vi "输入数据解析.vi"(0 "单个参数补充":dbl, 1 "从板号":dbl=1.0, 2 "主板二维码":string="BNET01", 3 "从板二维码":string="BNET01", 5 "主板引用":refnum<vi>, 7 "从板引用":refnum<vi>, 9 "主板选项":string="三级故障阀值", 11 "枚举":enum16{"主板", "从板"}(ring), 12 "快换":bool caption="快换写入") -> (4 "输出数组":dbl[][](array[numeric]), 6 "数组长度":dbl[](array[numeric]), 8 "循环次数":i32, 10 "命令":u32, 14 "名称":string[](array[string]), 15 "命令序号":u32[](array[numeric]))   [LabVIEW 2013] (continued)
                n1310 = Build Array(w3277) -> (w3278:i32[])
              }
              frame 16 {
                # "SOH过低"
                n1311 = disable-structure shown="启用" {
                  disable-tunnel: [w3302 w3310] -> w3289
                  disable-tunnel: w3288 -> [w3299 _]
                  disable-tunnel: [w3291 w3310] -> w3287
                  frame Disabled {
                    n1312 = Unbundle By Name(w3299) -> ("SOH过低"=w3298:dbl)
                    n1313 = call "输入分辨率计算-EV05.vi"("1字节?"=FALSE, "数值"=w3298, "偏移量"=0.0, "分辨率"=0.1) -> ("低字节"=w3300:dbl, "高字节1"=w3301:dbl)  [unwired: 1 in, 5 out]
                    n1314 = call "二进制解析-8.6.vi"("索引"=4, "数值"=w3301) -> ("低位子数组"=w3304:i32[])  [unwired: 3 out]
                    n1315 = call "二进制解析-8.6.vi"("索引"=4, "数值"=w3300) -> ("低位子数组"=w3293:i32[], "高位子数组"=w3303:i32[])  [unwired: 2 out]
                    n1316 = call "二进制解析-8.6.vi"("索引"=4, "数值"=0) -> ("低位子数组"=w3294:i32[])  [unwired: 3 out]
                    n1317 = Insert Into Array(array=w3304, new element=w3303) -> (w3297:i32[])  [unwired: 1 in]
                    n1318 = Insert Into Array(array=w3293, new element=w3294) -> (w3292:i32[])  [unwired: 1 in]
                    n1319 = call "数值二进制转十进制-8.6.vi"("子数组"=w3297) -> ("十进制数值"=w3302:i32)  [unwired: 4 out]
                    n1320 = call "数值二进制转十进制-8.6.vi"("子数组"=w3292) -> ("十进制数值"=w3291:i32)  [unwired: 4 out]
                  }
                  frame Enabled {
                    w3310 = 255 ("高字节1")
                  }
                }
                n1321 = Build Array(w3289, w3287) -> (w3290:i32[])
              }
            }
            n1322 = Insert Into Array(array=w3094, new element=w3095) -> (w3093:dbl[])  [unwired: 1 in]
          }
          n1323 = Build Array(w3090) -> (w3089:dbl[][])
          n1324 = Build Array("一级故障阀值") -> (w3080:string[])
        }
        frame "温度过低(2)" {
          n1325 = Unbundle By Name(w3316) -> ("一级故障 2"=w3317:refnum<vi>)
          n1326 = property class="Clust (严格)"(reference=w3317) -> ("Value"=w3315:T4)  [unwired: 1 in, 2 out]
          n1327 = for {
            N: 17 -> [_]
            tunnel: w3315 -> [w3327]
            shift-right: [w3324] -> w3321
            shift-left: dbl[] [] -> [w3325]
            i -> [w3328]
            n1328 = case shown="13" w3328 {
              tunnel: w3327 -> [w3329 w3340 w3351 w3361 w3371 w3381 w3393 w3405 w3417 w3429 w3441 w3453 w3467 w3489 w3501 w3510 w3519]
              tunnel: [w3330 w3341 w3352 w3362 w3372 w3383 w3395 w3407 w3419 w3431 w3443 w3454 w3476 w3492 w3500 w3509 w3521] -> w3326
              frame 0, Default {
                # "总电压过高"
                n1329 = disable-structure shown="启用" {
                  disable-tunnel: [w3336 w3339] -> w3332
                  disable-tunnel: [w3335 w3339] -> w3331
                  disable-tunnel: w3329 -> [w3334 _]
                  frame Disabled {
                    n1330 = Unbundle By Name(w3334) -> ("总电压过高"=w3333:dbl)
                    n1331 = call "输入分辨率计算-EV05.vi"("1字节?"=FALSE, "数值"=w3333, "分辨率"=0.1) -> ("低字节"=w3336:dbl, "高字节1"=w3335:dbl)  [unwired: 2 in, 5 out]
                  }
                  frame Enabled {
                    w3339 = 255 ("高字节1")
                  }
                }
                n1332 = Build Array(w3331, w3332) -> (w3330:i32[])
              }
              frame 1 {
                # "总电压过低"
                n1333 = disable-structure shown="启用" {
                  disable-tunnel: [w3347 w3350] -> w3343
                  disable-tunnel: [w3346 w3350] -> w3342
                  disable-tunnel: w3340 -> [w3345 _]
                  frame Disabled {
                    n1334 = Unbundle By Name(w3345) -> ("总电压过低"=w3344:dbl)
                    n1335 = call "输入分辨率计算-EV05.vi"("1字节?"=FALSE, "数值"=w3344, "分辨率"=0.1) -> ("低字节"=w3347:dbl, "高字节1"=w3346:dbl)  [unwired: 2 in, 5 out]
                  }
                  frame Enabled {
                    w3350 = 255 ("高字节1")
                  }
                }
                n1336 = Build Array(w3342, w3343) -> (w3341:i32[])
              }
              frame 2 {
                # "温度过高"
                n1337 = disable-structure shown="启用" {
                  disable-tunnel: [w3357 255 ("高字节1")] -> w3353
                  disable-tunnel: w3351 -> [w3355 _]
                  frame Disabled {
                    n1338 = Unbundle By Name(w3355) -> ("温度过高"=w3354:dbl)
                    n1339 = call "输入分辨率计算-EV05.vi"("1字节?"=TRUE, "数值"=w3354, "偏移量"=-40.0, "分辨率"=1.0) -> ("高字节1"=w3357:dbl)  [unwired: 1 in, 6 out]
                  }
                  frame Enabled {
                  }
                }
                n1340 = Build Array(w3353) -> (w3352:i32[])
              }
              frame 3 {
                # "温度过低"
                n1341 = disable-structure shown="启用" {
                  disable-tunnel: [w3367 255 ("高字节1")] -> w3363
                  disable-tunnel: w3361 -> [w3365 _]
                  frame Enabled {
                    n1342 = Unbundle By Name(w3365) -> ("温度过低"=w3364:dbl)
                    n1343 = call "输入分辨率计算-EV05.vi"("1字节?"=TRUE, "数值"=w3364, "偏移量"=-40.0, "分辨率"=1.0) -> ("高字节1"=w3367:dbl)  [unwired: 1 in, 6 out]
                  }
                  frame Disabled {
                  }
                }
                n1344 = Build Array(w3363) -> (w3362:dbl[])
              }
              frame 4 {
                # "整组温度不均衡"
                n1345 = disable-structure shown="启用" {
                  disable-tunnel: [w3377 255 ("高字节1")] -> w3373
                  disable-tunnel: w3371 -> [w3375 _]
                  frame Disabled {
                    n1346 = Unbundle By Name(w3375) -> ("整组温度不均衡"=w3374:dbl)
                    n1347 = call "输入分辨率计算-EV05.vi"("1字节?"=TRUE, "数值"=w3374, "偏移量"=0.0, "分辨率"=1.0) -> ("高字节1"=w3377:dbl)  [unwired: 1 in, 6 out]
                  }
                  frame Enabled {
                  }
                }
                n1348 = Build Array(w3373) -> (w3372:i32[])
              }
              frame 5 {
                # "单组电压不均衡"
                n1349 = disable-structure shown="启用" {
                  disable-tunnel: [w3389 w3392] -> w3384
                  disable-tunnel: [w3387 w3392] -> w3382
                  disable-tunnel: w3381 -> [w3386 _]
                  frame Disabled {
                    n1350 = Unbundle By Name(w3386) -> ("单组电压不均衡"=w3385:dbl)
                    n1351 = call "输入分辨率计算-EV05.vi"("1字节?"=FALSE, "数值"=w3385, "偏移量"=0.0, "分辨率"=0.001) -> ("低字节"=w3387:dbl, "高字节1"=w3389:dbl)  [unwired: 1 in, 5 out]
                  }
                  frame Enabled {
                    w3392 = 255 ("高字节1")
                  }
                }
                n1352 = Build Array(w3384, w3382) -> (w3383:i32[])
              }
              frame 6 {
                # "整组电压不均衡"
                n1353 = disable-structure shown="启用" {
                  disable-tunnel: [w3401 w3404] -> w3396
                  disable-tunnel: [w3399 w3404] -> w3394
                  disable-tunnel: w3393 -> [w3398 _]
                  frame Disabled {
                    n1354 = Unbundle By Name(w3398) -> ("整组电压不均衡"=w3397:dbl)
                    n1355 = call "输入分辨率计算-EV05.vi"("1字节?"=FALSE, "数值"=w3397, "偏移量"=0.0, "分辨率"=0.001) -> ("低字节"=w3399:dbl, "高字节1"=w3401:dbl)  [unwired: 1 in, 5 out]
                  }
                  frame Enabled {
                    w3404 = 255 ("高字节1")
                  }
                }
                n1356 = Build Array(w3396, w3394) -> (w3395:i32[])
              }
              frame 7 {
                # "单体电压过高"
                n1357 = disable-structure shown="启用" {
                  disable-tunnel: [w3413 w3416] -> w3408
                  disable-tunnel: [w3411 w3416] -> w3406
                  disable-tunnel: w3405 -> [w3410 _]
                  frame Disabled {
                    n1358 = Unbundle By Name(w3410) -> ("单体电压过高"=w3409:dbl)
                    n1359 = call "输入分辨率计算-EV05.vi"("1字节?"=FALSE, "数值"=w3409, "偏移量"=0.0, "分辨率"=0.001) -> ("低字节"=w3411:dbl, "高字节1"=w3413:dbl)  [unwired: 1 in, 5 out]
                  }
                  frame Enabled {
                    w3416 = 255 ("高字节1")
                  }
                }
                n1360 = Build Array(w3408, w3406) -> (w3407:i32[])
              }
              frame 8 {
                # "单体电压过低"
                n1361 = disable-structure shown="启用" {
                  disable-tunnel: [w3425 w3428] -> w3420
                  disable-tunnel: [w3423 w3428] -> w3418
                  disable-tunnel: w3417 -> [w3422 _]
                  frame Disabled {
                    n1362 = Unbundle By Name(w3422) -> ("单体电压过低"=w3421:dbl)
                    n1363 = call "输入分辨率计算-EV05.vi"("1字节?"=FALSE, "数值"=w3421, "偏移量"=0.0, "分辨率"=0.001) -> ("低字节"=w3423:dbl, "高字节1"=w3425:dbl)  [unwired: 1 in, 5 out]
                  }
                  frame Enabled {
                    w3428 = 255 ("高字节1")
                  }
                }
                n1364 = Build Array(w3420, w3418) -> (w3419:i32[])
              }
              frame 9 {
                # "充电电流过高"
                n1365 = disable-structure shown="启用" {
                  disable-tunnel: [w3437 w3440] -> w3432
                  disable-tunnel: [w3435 w3440] -> w3430
                  disable-tunnel: w3429 -> [w3434 _]
                  frame Disabled {
                    n1366 = Unbundle By Name(w3434) -> ("充电电流过高"=w3433:dbl)
                    n1367 = call "输入分辨率计算-EV05.vi"("1字节?"=FALSE, "数值"=w3433, "偏移量"=-3000.0, "分辨率"=0.1) -> ("低字节"=w3435:dbl, "高字节1"=w3437:dbl)  [unwired: 1 in, 5 out]
                  }
                  frame Enabled {
                    w3440 = 255 ("高字节1")
                  }
                }
                n1368 = Build Array(w3432, w3430) -> (w3431:i32[])
              }
              frame 10 {
                # "放电电流过高"
                n1369 = disable-structure shown="启用" {
                  disable-tunnel: [w3449 w3452] -> w3444
                  disable-tunnel: [w3447 w3452] -> w3442
                  disable-tunnel: w3441 -> [w3446 _]
                  frame Disabled {
                    n1370 = Unbundle By Name(w3446) -> ("放电电流过高"=w3445:dbl)
                    n1371 = call "输入分辨率计算-EV05.vi"("1字节?"=FALSE, "数值"=w3445, "偏移量"=-3000.0, "分辨率"=0.1) -> ("低字节"=w3447:dbl, "高字节1"=w3449:dbl)  [unwired: 1 in, 5 out]
                  }
                  frame Enabled {
                    w3452 = 255 ("高字节1")
                  }
                }
                n1372 = Build Array(w3444, w3442) -> (w3443:i32[])
              }
              frame 11 {
                # "单组温度不均衡"
                n1373 = disable-structure shown="启用" {
                  disable-tunnel: [w3459 255 ("高字节1")] -> w3455
                  disable-tunnel: w3453 -> [w3457 _]
                  frame Disabled {
                    n1374 = Unbundle By Name(w3457) -> ("单组温度不均衡"=w3456:dbl)
                    n1375 = call "输入分辨率计算-EV05.vi"("1字节?"=TRUE, "数值"=w3456, "偏移量"=0.0, "分辨率"=1.0) -> ("高字节1"=w3459:dbl)  [unwired: 1 in, 6 out]
                  }
                  frame Enabled {
                  }
                }
                n1376 = Build Array(w3455) -> (w3454:i32[])
              }
              frame 12 {
                # "SOC过高"
                n1377 = Unbundle By Name(w3467) -> ("SOC过高"=w3466:dbl)
                n1378 = call "输入分辨率计算-EV05.vi"("1字节?"=FALSE, "数值"=w3466, "偏移量"=0.0, "分辨率"=0.1) -> ("低字节"=w3468:dbl, "高字节1"=w3469:dbl)  [unwired: 1 in, 5 out]
                n1379 = call "二进制解析-8.6.vi"("索引"=4, "数值"=w3469) -> ("低位子数组"=w3472:i32[])  [unwired: 3 out]
                n1380 = call "二进制解析-8.6.vi"("索引"=4, "数值"=w3468) -> ("低位子数组"=w3464:i32[], "高位子数组"=w3471:i32[])  [unwired: 2 out]
                n1381 = Insert Into Array(array=w3472, new element=w3471) -> (w3470:i32[])  [unwired: 1 in]
                n1382 = call "数值二进制转十进制-8.6.vi"("子数组"=w3470) -> ("十进制数值"=w3465:i32)  [unwired: 4 out]
                n1383 = disable-structure shown="启用" {
                  disable-tunnel: w3465 -> [w3480 _]
                  disable-tunnel: [w3480 255 ("高字节1")] -> w3463
                  disable-tunnel: [w3479 i32[] [] ("低位子数组 21")] -> _
                  disable-tunnel: w3464 -> [w3479 _]
                  frame Disabled {
                  }
                  frame Enabled {
                  }
                }
                n1384 = Build Array(w3463, w3463) -> (w3476:i32[])
              }
              frame 13 {
                # "SOC过低"
                n1385 = Unbundle By Name(w3489) -> ("SOC过低"=w3488:dbl)
                n1386 = call "输入分辨率计算-EV05.vi"("1字节?"=FALSE, "数值"=w3488, "偏移量"=0.0, "分辨率"=0.1) -> ("低字节"=w3486:dbl, "高字节1"=w3487:dbl)  [unwired: 1 in, 5 out]
                n1387 = call "二进制解析-8.6.vi"("索引"=4, "数值"=w3487) -> ("低位子数组"=w3484:i32[])  [unwired: 3 out]
                n1388 = disable-structure shown="启用" {
                  disable-tunnel: w3486 -> [w3496 _]
                  disable-tunnel: [w3496 255 ("高字节1")] -> w3485
                  disable-tunnel: w3484 -> [w3495 _]
                  disable-tunnel: [_ 255 ("高字节1")] -> w3483
                  frame Disabled {
                    (unwired) i32[] [] ("低位子数组 4")
                  }
                  frame Enabled {
                  }
                }
                n1389 = Build Array(w3483, w3485) -> (w3492:i32[])
              }
              frame 14 {
                # "内阻过大"
                n1390 = disable-structure shown="启用" {
                  disable-tunnel: w3501 -> [w3506 _]
                  disable-tunnel: [w3502 255 ("高字节1")] -> w3499
                  frame Disabled {
                    n1391 = Unbundle By Name(w3506) -> ("内阻过大"=w3505:dbl)
                    n1392 = call "输入分辨率计算-EV05.vi"("1字节?"=TRUE, "数值"=w3505, "分辨率"=0.1) -> ("高字节1"=w3502:dbl)  [unwired: 2 in, 6 out]
                  }
                  frame Enabled {
                  }
                }
                n1393 = Build Array(w3499) -> (w3500:i32[])
              }
              frame 15 {
                # "极柱温度过高"
                n1394 = disable-structure shown="启用" {
                  disable-tunnel: w3510 -> [w3516 _]
                  disable-tunnel: [w3512 255 ("高字节1")] -> w3508
                  frame Disabled {
                    n1395 = Unbundle By Name(w3516) -> ("极柱温度过高"=w3515:dbl)
                    n1396 = call "输入分辨率计算-EV05.vi"("1字节?"=TRUE, "数值"=w3515, "偏移量"=-40.0, "分辨率"=1.0) -> ("高字节1"=w3512:dbl)  [unwired: 1 in, 6 out]
                  }
                  frame Enabled {
                  }
                }
                n1397 = Build Array(w3508) -> (w3509:i32[])
              }
              frame 16 {
                # "SOH过低"
                n1398 = disable-structure shown="启用" {
                  disable-tunnel: [w3533 w3541] -> w3520
                  disable-tunnel: w3519 -> [w3530 _]
                  disable-tunnel: [w3522 w3541] -> w3518
                  frame Disabled {
                    n1399 = Unbundle By Name(w3530) -> ("SOH过低"=w3529:dbl)
                    n1400 = call "输入分辨率计算-EV05.vi"("1字节?"=FALSE, "数值"=w3529, "偏移量"=0.0, "分辨率"=0.1) -> ("低字节"=w3531:dbl, "高字节1"=w3532:dbl)  [unwired: 1 in, 5 out]
                    n1401 = call "二进制解析-8.6.vi"("索引"=4, "数值"=w3532) -> ("低位子数组"=w3535:i32[])  [unwired: 3 out]
                    n1402 = call "二进制解析-8.6.vi"("索引"=4, "数值"=w3531) -> ("低位子数组"=w3524:i32[], "高位子数组"=w3534:i32[])  [unwired: 2 out]
                    n1403 = call "二进制解析-8.6.vi"("索引"=4, "数值"=0) -> ("低位子数组"=w3525:i32[])  [unwired: 3 out]
                    n1404 = Insert Into Array(array=w3535, new element=w3534) -> (w3528:i32[])  [unwired: 1 in]
                    n1405 = Insert Into Array(array=w3524, new element=w3525) -> (w3523:i32[])  [unwired: 1 in]
                    n1406 = call "数值二进制转十进制-8.6.vi"("子数组"=w3528) -> ("十进制数值"=w3533:i32)  [unwired: 4 out]
                    n1407 = call "数值二进制转十进制-8.6.vi"("子数组"=w3523) -> ("十进制数值"=w3522:i32)  [unwired: 4 out]
                  }
                  frame Enabled {
                    w3541 = 255 ("高字节1")
                  }
                }
                n1408 = Build Array(w3520, w3518) -> (w3521:i32[])
              }
            }
            n1409 = Insert Into Array(array=w3325, new element=w3326) -> (w3324:dbl[])  [unwired: 1 in]
          }
          n1410 = Build Array(w3321) -> (w3320:dbl[][])
          n1411 = Build Array("二级故障阀值") -> (w3311:string[])
        }
        frame "温度过低(3)" {
          n1412 = Unbundle By Name(w3547) -> ("一级故障 3"=w3548:refnum<vi>)
          n1413 = property class="Clust (严格)"(reference=w3548) -> ("Value"=w3546:T4)  [unwired: 1 in, 2 out]
          n1414 = for {
            N: 17 -> [_]
            tunnel: w3546 -> [w3558]
            shift-right: [w3555] -> w3552
            shift-left: dbl[] [] -> [w3556]
            i -> [w3559]
            n1415 = case shown="13" w3559 {
              tunnel: w3558 -> [w3560 w3571 w3582 w3592 w3602 w3612 w3624 w3636 w3648 w3660 w3672 w3684 w3698 w3720 w3732 w3741 w3750]
              tunnel: [w3561 w3572 w3583 w3593 w3603 w3614 w3626 w3638 w3650 w3662 w3674 w3685 w3707 w3723 w3731 w3740 w3752] -> w3557
              frame 0, Default {
                # "总电压过高"
                n1416 = disable-structure shown="启用" {
                  disable-tunnel: [w3567 w3570] -> w3563
                  disable-tunnel: [w3566 w3570] -> w3562
                  disable-tunnel: w3560 -> [w3565 _]
                  frame Disabled {
                    n1417 = Unbundle By Name(w3565) -> ("总电压过高"=w3564:dbl)
                    n1418 = call "输入分辨率计算-EV05.vi"("1字节?"=FALSE, "数值"=w3564, "分辨率"=0.1) -> ("低字节"=w3567:dbl, "高字节1"=w3566:dbl)  [unwired: 2 in, 5 out]
                  }
                  frame Enabled {
                    w3570 = 255 ("高字节1")
                  }
                }
                n1419 = Build Array(w3562, w3563) -> (w3561:i32[])
              }
              frame 1 {
                # "总电压过低"
                n1420 = disable-structure shown="启用" {
                  disable-tunnel: [w3578 w3581] -> w3574
                  disable-tunnel: [w3577 w3581] -> w3573
                  disable-tunnel: w3571 -> [w3576 _]
                  frame Disabled {
                    n1421 = Unbundle By Name(w3576) -> ("总电压过低"=w3575:dbl)
                    n1422 = call "输入分辨率计算-EV05.vi"("1字节?"=FALSE, "数值"=w3575, "分辨率"=0.1) -> ("低字节"=w3578:dbl, "高字节1"=w3577:dbl)  [unwired: 2 in, 5 out]
                  }
                  frame Enabled {
                    w3581 = 255 ("高字节1")
                  }
                }
                n1423 = Build Array(w3573, w3574) -> (w3572:i32[])
              }
              frame 2 {
                # "温度过高"
                n1424 = disable-structure shown="启用" {
                  disable-tunnel: [w3588 255 ("高字节1")] -> w3584
                  disable-tunnel: w3582 -> [w3586 _]
                  frame Disabled {
                    n1425 = Unbundle By Name(w3586) -> ("温度过高"=w3585:dbl)
                    n1426 = call "输入分辨率计算-EV05.vi"("1字节?"=TRUE, "数值"=w3585, "偏移量"=-40.0, "分辨率"=1.0) -> ("高字节1"=w3588:dbl)  [unwired: 1 in, 6 out]
                  }
                  frame Enabled {
                  }
                }
                n1427 = Build Array(w3584) -> (w3583:i32[])
              }
              frame 3 {
                # "温度过低"
                n1428 = disable-structure shown="启用" {
                  disable-tunnel: [w3598 255 ("高字节1")] -> w3594
                  disable-tunnel: w3592 -> [w3596 _]
                  frame Enabled {
                    n1429 = Unbundle By Name(w3596) -> ("温度过低"=w3595:dbl)
                    n1430 = call "输入分辨率计算-EV05.vi"("1字节?"=TRUE, "数值"=w3595, "偏移量"=-40.0, "分辨率"=1.0) -> ("高字节1"=w3598:dbl)  [unwired: 1 in, 6 out]
                  }
                  frame Disabled {
                  }
                }
                n1431 = Build Array(w3594) -> (w3593:dbl[])
              }
              frame 4 {
                # "整组温度不均衡"
                n1432 = disable-structure shown="启用" {
                  disable-tunnel: [w3608 255 ("高字节1")] -> w3604
                  disable-tunnel: w3602 -> [w3606 _]
                  frame Disabled {
                    n1433 = Unbundle By Name(w3606) -> ("整组温度不均衡"=w3605:dbl)
                    n1434 = call "输入分辨率计算-EV05.vi"("1字节?"=TRUE, "数值"=w3605, "偏移量"=0.0, "分辨率"=1.0) -> ("高字节1"=w3608:dbl)  [unwired: 1 in, 6 out]
                  }
                  frame Enabled {
                  }
                }
                n1435 = Build Array(w3604) -> (w3603:i32[])
              }
              frame 5 {
                # "单组电压不均衡"
                n1436 = disable-structure shown="启用" {
                  disable-tunnel: [w3620 w3623] -> w3615
                  disable-tunnel: [w3618 w3623] -> w3613
                  disable-tunnel: w3612 -> [w3617 _]
                  frame Disabled {
                    n1437 = Unbundle By Name(w3617) -> ("单组电压不均衡"=w3616:dbl)
                    n1438 = call "输入分辨率计算-EV05.vi"("1字节?"=FALSE, "数值"=w3616, "偏移量"=0.0, "分辨率"=0.001) -> ("低字节"=w3618:dbl, "高字节1"=w3620:dbl)  [unwired: 1 in, 5 out]
                  }
                  frame Enabled {
                    w3623 = 255 ("高字节1")
                  }
                }
                n1439 = Build Array(w3615, w3613) -> (w3614:i32[])
              }
              frame 6 {
                # "整组电压不均衡"
                n1440 = disable-structure shown="启用" {
                  disable-tunnel: [w3632 w3635] -> w3627
                  disable-tunnel: [w3630 w3635] -> w3625
                  disable-tunnel: w3624 -> [w3629 _]
                  frame Disabled {
                    n1441 = Unbundle By Name(w3629) -> ("整组电压不均衡"=w3628:dbl)
                    n1442 = call "输入分辨率计算-EV05.vi"("1字节?"=FALSE, "数值"=w3628, "偏移量"=0.0, "分辨率"=0.001) -> ("低字节"=w3630:dbl, "高字节1"=w3632:dbl)  [unwired: 1 in, 5 out]
                  }
                  frame Enabled {
                    w3635 = 255 ("高字节1")
                  }
                }
                n1443 = Build Array(w3627, w3625) -> (w3626:i32[])
              }
              frame 7 {
                # "单体电压过高"
                n1444 = disable-structure shown="启用" {
                  disable-tunnel: [w3644 w3647] -> w3639
                  disable-tunnel: [w3642 w3647] -> w3637
                  disable-tunnel: w3636 -> [w3641 _]
                  frame Disabled {
                    n1445 = Unbundle By Name(w3641) -> ("单体电压过高"=w3640:dbl)
                    n1446 = call "输入分辨率计算-EV05.vi"("1字节?"=FALSE, "数值"=w3640, "偏移量"=0.0, "分辨率"=0.001) -> ("低字节"=w3642:dbl, "高字节1"=w3644:dbl)  [unwired: 1 in, 5 out]
                  }
                  frame Enabled {
                    w3647 = 255 ("高字节1")
                  }
                }
                n1447 = Build Array(w3639, w3637) -> (w3638:i32[])
              }
              frame 8 {
                # "单体电压过低"
                n1448 = disable-structure shown="启用" {
                  disable-tunnel: [w3656 w3659] -> w3651
                  disable-tunnel: [w3654 w3659] -> w3649
                  disable-tunnel: w3648 -> [w3653 _]
                  frame Disabled {
                    n1449 = Unbundle By Name(w3653) -> ("单体电压过低"=w3652:dbl)
                    n1450 = call "输入分辨率计算-EV05.vi"("1字节?"=FALSE, "数值"=w3652, "偏移量"=0.0, "分辨率"=0.001) -> ("低字节"=w3654:dbl, "高字节1"=w3656:dbl)  [unwired: 1 in, 5 out]
                  }
                  frame Enabled {
                    w3659 = 255 ("高字节1")
                  }
                }
                n1451 = Build Array(w3651, w3649) -> (w3650:i32[])
              }
              frame 9 {
                # "充电电流过高"
                n1452 = disable-structure shown="启用" {
                  disable-tunnel: [w3668 w3671] -> w3663
                  disable-tunnel: [w3666 w3671] -> w3661
                  disable-tunnel: w3660 -> [w3665 _]
                  frame Disabled {
                    n1453 = Unbundle By Name(w3665) -> ("充电电流过高"=w3664:dbl)
                    n1454 = call "输入分辨率计算-EV05.vi"("1字节?"=FALSE, "数值"=w3664, "偏移量"=-3000.0, "分辨率"=0.1) -> ("低字节"=w3666:dbl, "高字节1"=w3668:dbl)  [unwired: 1 in, 5 out]
                  }
                  frame Enabled {
                    w3671 = 255 ("高字节1")
                  }
                }
                n1455 = Build Array(w3663, w3661) -> (w3662:i32[])
              }
              frame 10 {
                # "放电电流过高"
                n1456 = disable-structure shown="启用" {
                  disable-tunnel: [w3680 w3683] -> w3675
                  disable-tunnel: [w3678 w3683] -> w3673
                  disable-tunnel: w3672 -> [w3677 _]
                  frame Disabled {
                    n1457 = Unbundle By Name(w3677) -> ("放电电流过高"=w3676:dbl)
                    n1458 = call "输入分辨率计算-EV05.vi"("1字节?"=FALSE, "数值"=w3676, "偏移量"=-3000.0, "分辨率"=0.1) -> ("低字节"=w3678:dbl, "高字节1"=w3680:dbl)  [unwired: 1 in, 5 out]
                  }
                  frame Enabled {
                    w3683 = 255 ("高字节1")
                  }
                }
                n1459 = Build Array(w3675, w3673) -> (w3674:i32[])
              }
              frame 11 {
                # "单组温度不均衡"
                n1460 = disable-structure shown="启用" {
                  disable-tunnel: [w3690 255 ("高字节1")] -> w3686
                  disable-tunnel: w3684 -> [w3688 _]
                  frame Disabled {
                    n1461 = Unbundle By Name(w3688) -> ("单组温度不均衡"=w3687:dbl)
                    n1462 = call "输入分辨率计算-EV05.vi"("1字节?"=TRUE, "数值"=w3687, "偏移量"=0.0, "分辨率"=1.0) -> ("高字节1"=w3690:dbl)  [unwired: 1 in, 6 out]
                  }
                  frame Enabled {
                  }
                }
                n1463 = Build Array(w3686) -> (w3685:i32[])
              }
              frame 12 {
                # "SOC过高"
                n1464 = Unbundle By Name(w3698) -> ("SOC过高"=w3697:dbl)
                n1465 = call "输入分辨率计算-EV05.vi"("1字节?"=FALSE, "数值"=w3697, "偏移量"=0.0, "分辨率"=0.1) -> ("低字节"=w3699:dbl, "高字节1"=w3700:dbl)  [unwired: 1 in, 5 out]
                n1466 = call "二进制解析-8.6.vi"("索引"=4, "数值"=w3700) -> ("低位子数组"=w3703:i32[])  [unwired: 3 out]
                n1467 = call "二进制解析-8.6.vi"("索引"=4, "数值"=w3699) -> ("低位子数组"=w3695:i32[], "高位子数组"=w3702:i32[])  [unwired: 2 out]
                n1468 = Insert Into Array(array=w3703, new element=w3702) -> (w3701:i32[])  [unwired: 1 in]
                n1469 = call "数值二进制转十进制-8.6.vi"("子数组"=w3701) -> ("十进制数值"=w3696:i32)  [unwired: 4 out]
                n1470 = disable-structure shown="启用" {
                  disable-tunnel: w3696 -> [w3711 _]
                  disable-tunnel: [w3711 255 ("高字节1")] -> w3694
                  disable-tunnel: [w3710 i32[] [] ("低位子数组 21")] -> _
                  disable-tunnel: w3695 -> [w3710 _]
                  frame Disabled {
                  }
                  frame Enabled {
                  }
                }
                n1471 = Build Array(w3694, w3694) -> (w3707:i32[])
              }
              frame 13 {
                # "SOC过低"
                n1472 = Unbundle By Name(w3720) -> ("SOC过低"=w3719:dbl)
                n1473 = call "输入分辨率计算-EV05.vi"("1字节?"=FALSE, "数值"=w3719, "偏移量"=0.0, "分辨率"=0.1) -> ("低字节"=w3717:dbl, "高字节1"=w3718:dbl)  [unwired: 1 in, 5 out]
                n1474 = call "二进制解析-8.6.vi"("索引"=4, "数值"=w3718) -> ("低位子数组"=w3715:i32[])  [unwired: 3 out]
                n1475 = disable-structure shown="启用" {
                  disable-tunnel: w3717 -> [w3727 _]
                  disable-tunnel: [w3727 255 ("高字节1")] -> w3716
                  disable-tunnel: w3715 -> [w3726 _]
                  disable-tunnel: [_ 255 ("高字节1")] -> w3714
                  frame Disabled {
                    (unwired) i32[] [] ("低位子数组 4")
                  }
                  frame Enabled {
                  }
                }
                n1476 = Build Array(w3714, w3716) -> (w3723:i32[])
              }
              frame 14 {
                # "内阻过大"
                n1477 = disable-structure shown="启用" {
                  disable-tunnel: w3732 -> [w3737 _]
                  disable-tunnel: [w3733 255 ("高字节1")] -> w3730
                  frame Disabled {
                    n1478 = Unbundle By Name(w3737) -> ("内阻过大"=w3736:dbl)
                    n1479 = call "输入分辨率计算-EV05.vi"("1字节?"=TRUE, "数值"=w3736, "分辨率"=0.1) -> ("高字节1"=w3733:dbl)  [unwired: 2 in, 6 out]
                  }
                  frame Enabled {
                  }
                }
                n1480 = Build Array(w3730) -> (w3731:i32[])
              }
              frame 15 {
                # "极柱温度过高"
                n1481 = disable-structure shown="启用" {
                  disable-tunnel: w3741 -> [w3747 _]
                  disable-tunnel: [w3743 255 ("高字节1")] -> w3739
                  frame Disabled {
                    n1482 = Unbundle By Name(w3747) -> ("极柱温度过高"=w3746:dbl)
                    n1483 = call "输入分辨率计算-EV05.vi"("1字节?"=TRUE, "数值"=w3746, "偏移量"=-40.0, "分辨率"=1.0) -> ("高字节1"=w3743:dbl)  [unwired: 1 in, 6 out]
                  }
                  frame Enabled {
                  }
                }
                n1484 = Build Array(w3739) -> (w3740:i32[])
              }
              frame 16 {
                # "SOH过低"
                n1485 = disable-structure shown="启用" {
                  disable-tunnel: [w3764 w3772] -> w3751
                  disable-tunnel: w3750 -> [w3761 _]
                  disable-tunnel: [w3753 w3772] -> w3749
                  frame Disabled {
                    n1486 = Unbundle By Name(w3761) -> ("SOH过低"=w3760:dbl)
                    n1487 = call "输入分辨率计算-EV05.vi"("1字节?"=FALSE, "数值"=w3760, "偏移量"=0.0, "分辨率"=0.1) -> ("低字节"=w3762:dbl, "高字节1"=w3763:dbl)  [unwired: 1 in, 5 out]
                    n1488 = call "二进制解析-8.6.vi"("索引"=4, "数值"=w3763) -> ("低位子数组"=w3766:i32[])  [unwired: 3 out]
                    n1489 = call "二进制解析-8.6.vi"("索引"=4, "数值"=w3762) -> ("低位子数组"=w3755:i32[], "高位子数组"=w3765:i32[])  [unwired: 2 out]
                    n1490 = call "二进制解析-8.6.vi"("索引"=4, "数值"=0) -> ("低位子数组"=w3756:i32[])  [unwired: 3 out]
                    n1491 = Insert Into Array(array=w3766, new element=w3765) -> (w3759:i32[])  [unwired: 1 in]
                    n1492 = Insert Into Array(array=w3755, new element=w3756) -> (w3754:i32[])  [unwired: 1 in]
                    n1493 = call "数值二进制转十进制-8.6.vi"("子数组"=w3759) -> ("十进制数值"=w3764:i32)  [unwired: 4 out]
                    n1494 = call "数值二进制转十进制-8.6.vi"("子数组"=w3754) -> ("十进制数值"=w3753:i32)  [unwired: 4 out]
                  }
                  frame Enabled {
                    w3772 = 255 ("高字节1")
                  }
                }
                n1495 = Build Array(w3751, w3749) -> (w3752:i32[])
              }
            }
            n1496 = Insert Into Array(array=w3556, new element=w3557) -> (w3555:dbl[])  [unwired: 1 in]
          }
          n1497 = Build Array(w3552) -> (w3551:dbl[][])
          n1498 = Build Array("三级故障阀值") -> (w3542:string[])
        }
        frame "整组温度不均衡" {
          n1499 = Unbundle By Name(w3778) -> ("一级故障"=w3779:refnum<vi>)
          n1500 = property class="Clust (严格)"(reference=w3779) -> ("Value"=w3777:T4)  [unwired: 1 in, 2 out]
          n1501 = for {
            N: 17 -> [_]
            tunnel: w3777 -> [w3789]
            shift-right: [w3786] -> w3783
            shift-left: dbl[] [] -> [w3787]
            i -> [w3790]
            n1502 = case shown="11" w3790 {
              tunnel: w3789 -> [w3791 w3802 w3813 w3823 w3833 w3842 w3854 w3866 w3878 w3890 w3902 w3914 w3928 w3950 w3962 w3971 w3980]
              tunnel: [w3792 w3803 w3814 w3824 w3834 w3844 w3856 w3868 w3880 w3892 w3904 w3915 w3937 w3953 w3961 w3970 w3982] -> w3788
              frame 0, Default {
                # "总电压过高"
                n1503 = disable-structure shown="启用" {
                  disable-tunnel: [w3798 w3801] -> w3794
                  disable-tunnel: [w3797 w3801] -> w3793
                  disable-tunnel: w3791 -> [w3796 _]
                  frame Disabled {
                    n1504 = Unbundle By Name(w3796) -> ("总电压过高"=w3795:dbl)
                    n1505 = call "输入分辨率计算-EV05.vi"("1字节?"=FALSE, "数值"=w3795, "分辨率"=0.1) -> ("低字节"=w3798:dbl, "高字节1"=w3797:dbl)  [unwired: 2 in, 5 out]
                  }
                  frame Enabled {
                    w3801 = 255 ("高字节1")
                  }
                }
                n1506 = Build Array(w3793, w3794) -> (w3792:i32[])
              }
              frame 1 {
                # "总电压过低"
                n1507 = disable-structure shown="启用" {
                  disable-tunnel: [w3809 w3812] -> w3805
                  disable-tunnel: [w3808 w3812] -> w3804
                  disable-tunnel: w3802 -> [w3807 _]
                  frame Disabled {
                    n1508 = Unbundle By Name(w3807) -> ("总电压过低"=w3806:dbl)
                    n1509 = call "输入分辨率计算-EV05.vi"("1字节?"=FALSE, "数值"=w3806, "分辨率"=0.1) -> ("低字节"=w3809:dbl, "高字节1"=w3808:dbl)  [unwired: 2 in, 5 out]
                  }
                  frame Enabled {
                    w3812 = 255 ("高字节1")
                  }
                }
                n1510 = Build Array(w3804, w3805) -> (w3803:i32[])
              }
              frame 2 {
                # "温度过高"
                n1511 = disable-structure shown="启用" {
                  disable-tunnel: [w3819 255 ("高字节1")] -> w3815
                  disable-tunnel: w3813 -> [w3817 _]
                  frame Disabled {
                    n1512 = Unbundle By Name(w3817) -> ("温度过高"=w3816:dbl)
                    n1513 = call "输入分辨率计算-EV05.vi"("1字节?"=TRUE, "数值"=w3816, "偏移量"=-40.0, "分辨率"=1.0) -> ("高字节1"=w3819:dbl)  [unwired: 1 in, 6 out]
                  }
                  frame Enabled {
                  }
                }
                n1514 = Build Array(w3815) -> (w3814:i32[])
              }
              frame 3 {
                # "温度过低"
                n1515 = disable-structure shown="启用" {
                  disable-tunnel: [w3829 255 ("高字节1")] -> w3825
                  disable-tunnel: w3823 -> [w3827 _]
                  frame Disabled {
                    n1516 = Unbundle By Name(w3827) -> ("温度过低"=w3826:dbl)
                    n1517 = call "输入分辨率计算-EV05.vi"("1字节?"=TRUE, "数值"=w3826, "偏移量"=-40.0, "分辨率"=1.0) -> ("高字节1"=w3829:dbl)  [unwired: 1 in, 6 out]
                  }
                  frame Enabled {
                  }
                }
                n1518 = Build Array(w3825) -> (w3824:i32[])
              }
              frame 4 {
                # "整组温度不均衡"
                n1519 = disable-structure shown="启用" {
                  disable-tunnel: [w3838 255 ("高字节1")] -> w3835
                  disable-tunnel: w3833 -> [w3837 _]
                  frame Enabled {
                    n1520 = Unbundle By Name(w3837) -> ("整组温度不均衡"=w3836:dbl)
                    n1521 = call "输入分辨率计算-EV05.vi"("1字节?"=TRUE, "数值"=w3836, "分辨率"=1.0) -> ("高字节1"=w3838:dbl)  [unwired: 2 in, 6 out]
                  }
                  frame Disabled {
                  }
                }
                n1522 = Build Array(w3835) -> (w3834:dbl[])
              }
              frame 5 {
                # "单组电压不均衡"
                n1523 = disable-structure shown="启用" {
                  disable-tunnel: [w3850 w3853] -> w3845
                  disable-tunnel: [w3848 w3853] -> w3843
                  disable-tunnel: w3842 -> [w3847 _]
                  frame Disabled {
                    n1524 = Unbundle By Name(w3847) -> ("单组电压不均衡"=w3846:dbl)
                    n1525 = call "输入分辨率计算-EV05.vi"("1字节?"=FALSE, "数值"=w3846, "偏移量"=0.0, "分辨率"=0.001) -> ("低字节"=w3848:dbl, "高字节1"=w3850:dbl)  [unwired: 1 in, 5 out]
                  }
                  frame Enabled {
                    w3853 = 255 ("高字节1")
                  }
                }
                n1526 = Build Array(w3845, w3843) -> (w3844:i32[])
              }
              frame 6 {
                # "整组电压不均衡"
                n1527 = disable-structure shown="启用" {
                  disable-tunnel: [w3862 w3865] -> w3857
                  disable-tunnel: [w3860 w3865] -> w3855
                  disable-tunnel: w3854 -> [w3859 _]
                  frame Disabled {
                    n1528 = Unbundle By Name(w3859) -> ("整组电压不均衡"=w3858:dbl)
                    n1529 = call "输入分辨率计算-EV05.vi"("1字节?"=FALSE, "数值"=w3858, "偏移量"=0.0, "分辨率"=0.001) -> ("低字节"=w3860:dbl, "高字节1"=w3862:dbl)  [unwired: 1 in, 5 out]
                  }
                  frame Enabled {
                    w3865 = 255 ("高字节1")
                  }
                }
                n1530 = Build Array(w3857, w3855) -> (w3856:i32[])
              }
              frame 7 {
                # "单体电压过高"
                n1531 = disable-structure shown="启用" {
                  disable-tunnel: [w3874 w3877] -> w3869
                  disable-tunnel: [w3872 w3877] -> w3867
                  disable-tunnel: w3866 -> [w3871 _]
                  frame Disabled {
                    n1532 = Unbundle By Name(w3871) -> ("单体电压过高"=w3870:dbl)
                    n1533 = call "输入分辨率计算-EV05.vi"("1字节?"=FALSE, "数值"=w3870, "偏移量"=0.0, "分辨率"=0.001) -> ("低字节"=w3872:dbl, "高字节1"=w3874:dbl)  [unwired: 1 in, 5 out]
                  }
                  frame Enabled {
                    w3877 = 255 ("高字节1")
                  }
                }
                n1534 = Build Array(w3869, w3867) -> (w3868:i32[])
              }
              frame 8 {
                # "单体电压过低"
                n1535 = disable-structure shown="启用" {
                  disable-tunnel: [w3886 w3889] -> w3881
                  disable-tunnel: [w3884 w3889] -> w3879
                  disable-tunnel: w3878 -> [w3883 _]
                  frame Disabled {
                    n1536 = Unbundle By Name(w3883) -> ("单体电压过低"=w3882:dbl)
                    n1537 = call "输入分辨率计算-EV05.vi"("1字节?"=FALSE, "数值"=w3882, "偏移量"=0.0, "分辨率"=0.001) -> ("低字节"=w3884:dbl, "高字节1"=w3886:dbl)  [unwired: 1 in, 5 out]
                  }
                  frame Enabled {
                    w3889 = 255 ("高字节1")
                  }
                }
                n1538 = Build Array(w3881, w3879) -> (w3880:i32[])
              }
              frame 9 {
                # "充电电流过高"
                n1539 = disable-structure shown="启用" {
                  disable-tunnel: [w3898 w3901] -> w3893
                  disable-tunnel: [w3896 w3901] -> w3891
                  disable-tunnel: w3890 -> [w3895 _]
                  frame Disabled {
                    n1540 = Unbundle By Name(w3895) -> ("充电电流过高"=w3894:dbl)
                    n1541 = call "输入分辨率计算-EV05.vi"("1字节?"=FALSE, "数值"=w3894, "偏移量"=-3000.0, "分辨率"=0.1) -> ("低字节"=w3896:dbl, "高字节1"=w3898:dbl)  [unwired: 1 in, 5 out]
                  }
                  frame Enabled {
                    w3901 = 255 ("高字节1")
                  }
                }
                n1542 = Build Array(w3893, w3891) -> (w3892:i32[])
              }
              frame 10 {
                # "放电电流过高"
                n1543 = disable-structure shown="启用" {
                  disable-tunnel: [w3910 w3913] -> w3905
                  disable-tunnel: [w3908 w3913] -> w3903
                  disable-tunnel: w3902 -> [w3907 _]
                  frame Disabled {
                    n1544 = Unbundle By Name(w3907) -> ("放电电流过高"=w3906:dbl)
                    n1545 = call "输入分辨率计算-EV05.vi"("1字节?"=FALSE, "数值"=w3906, "偏移量"=-3000.0, "分辨率"=0.1) -> ("低字节"=w3908:dbl, "高字节1"=w3910:dbl)  [unwired: 1 in, 5 out]
                  }
                  frame Enabled {
                    w3913 = 255 ("高字节1")
                  }
                }
                n1546 = Build Array(w3905, w3903) -> (w3904:i32[])
              }
              frame 11 {
                # "单组温度不均衡"
                n1547 = disable-structure shown="启用" {
                  disable-tunnel: [w3920 255 ("高字节1")] -> w3916
                  disable-tunnel: w3914 -> [w3918 _]
                  frame Disabled {
                    n1548 = Unbundle By Name(w3918) -> ("单组温度不均衡"=w3917:dbl)
                    n1549 = call "输入分辨率计算-EV05.vi"("1字节?"=TRUE, "数值"=w3917, "偏移量"=0.0, "分辨率"=1.0) -> ("高字节1"=w3920:dbl)  [unwired: 1 in, 6 out]
                  }
                  frame Enabled {
                  }
                }
                n1550 = Build Array(w3916) -> (w3915:i32[])
              }
              frame 12 {
                # "SOC过高"
                n1551 = Unbundle By Name(w3928) -> ("SOC过高"=w3927:dbl)
                n1552 = call "输入分辨率计算-EV05.vi"("1字节?"=FALSE, "数值"=w3927, "偏移量"=0.0, "分辨率"=0.1) -> ("低字节"=w3929:dbl, "高字节1"=w3930:dbl)  [unwired: 1 in, 5 out]
                n1553 = call "二进制解析-8.6.vi"("索引"=4, "数值"=w3930) -> ("低位子数组"=w3933:i32[])  [unwired: 3 out]
                n1554 = call "二进制解析-8.6.vi"("索引"=4, "数值"=w3929) -> ("低位子数组"=w3925:i32[], "高位子数组"=w3932:i32[])  [unwired: 2 out]
                n1555 = Insert Into Array(array=w3933, new element=w3932) -> (w3931:i32[])  [unwired: 1 in]
                n1556 = call "数值二进制转十进制-8.6.vi"("子数组"=w3931) -> ("十进制数值"=w3926:i32)  [unwired: 4 out]
                n1557 = disable-structure shown="禁用" {
                  disable-tunnel: w3926 -> [w3941 _]
                  disable-tunnel: [w3941 255 ("高字节1")] -> w3924
                  disable-tunnel: [w3940 i32[] [] ("低位子数组 22")] -> _
                  disable-tunnel: w3925 -> [w3940 _]
                  frame Disabled {
                  }
                  frame Enabled {
                  }
                }
                n1558 = Build Array(w3924, w3924) -> (w3937:i32[])
              }
              frame 13 {
                # "SOC过低"
                n1559 = Unbundle By Name(w3950) -> ("SOC过低"=w3949:dbl)
                n1560 = call "输入分辨率计算-EV05.vi"("1字节?"=FALSE, "数值"=w3949, "偏移量"=0.0, "分辨率"=0.1) -> ("低字节"=w3947:dbl, "高字节1"=w3948:dbl)  [unwired: 1 in, 5 out]
                n1561 = call "二进制解析-8.6.vi"("索引"=4, "数值"=w3948) -> ("低位子数组"=w3945:i32[])  [unwired: 3 out]
                n1562 = disable-structure shown="启用" {
                  disable-tunnel: w3947 -> [w3957 _]
                  disable-tunnel: [w3957 255 ("高字节1")] -> w3946
                  disable-tunnel: w3945 -> [w3956 _]
                  disable-tunnel: [_ 255 ("高字节1")] -> w3944
                  frame Disabled {
                    (unwired) i32[] [] ("低位子数组 4")
                  }
                  frame Enabled {
                  }
                }
                n1563 = Build Array(w3944, w3946) -> (w3953:i32[])
              }
              frame 14 {
                # "内阻过大"
                n1564 = disable-structure shown="启用" {
                  disable-tunnel: w3962 -> [w3967 _]
                  disable-tunnel: [w3963 255 ("高字节1")] -> w3960
                  frame Disabled {
                    n1565 = Unbundle By Name(w3967) -> ("内阻过大"=w3966:dbl)
                    n1566 = call "输入分辨率计算-EV05.vi"("1字节?"=TRUE, "数值"=w3966, "分辨率"=0.1) -> ("高字节1"=w3963:dbl)  [unwired: 2 in, 6 out]
                  }
                  frame Enabled {
                  }
                }
                n1567 = Build Array(w3960) -> (w3961:i32[])
              }
              frame 15 {
                # "极柱温度过高"
                n1568 = disable-structure shown="启用" {
                  disable-tunnel: w3971 -> [w3977 _]
                  disable-tunnel: [w3973 255 ("高字节1")] -> w3969
                  frame Disabled {
                    n1569 = Unbundle By Name(w3977) -> ("极柱温度过高"=w3976:dbl)
                    n1570 = call "输入分辨率计算-EV05.vi"("1字节?"=TRUE, "数值"=w3976, "偏移量"=-40.0, "分辨率"=1.0) -> ("高字节1"=w3973:dbl)  [unwired: 1 in, 6 out]
                  }
                  frame Enabled {
                  }
                }
                n1571 = Build Array(w3969) -> (w3970:i32[])
              }
              frame 16 {
                # "SOH过低"
                n1572 = disable-structure shown="启用" {
                  disable-tunnel: [w3994 w4002] -> w3981
                  disable-tunnel: w3980 -> [w3991 _]
                  disable-tunnel: [w3983 w4002] -> w3979
                  frame Disabled {
                    n1573 = Unbundle By Name(w3991) -> ("SOH过低"=w3990:dbl)
                    n1574 = call "输入分辨率计算-EV05.vi"("1字节?"=FALSE, "数值"=w3990, "偏移量"=0.0, "分辨率"=0.1) -> ("低字节"=w3992:dbl, "高字节1"=w3993:dbl)  [unwired: 1 in, 5 out]
                    n1575 = call "二进制解析-8.6.vi"("索引"=4, "数值"=w3993) -> ("低位子数组"=w3996:i32[])  [unwired: 3 out]
                    n1576 = call "二进制解析-8.6.vi"("索引"=4, "数值"=w3992) -> ("低位子数组"=w3985:i32[], "高位子数组"=w3995:i32[])  [unwired: 2 out]
                    n1577 = call "二进制解析-8.6.vi"("索引"=4, "数值"=0) -> ("低位子数组"=w3986:i32[])  [unwired: 3 out]
                    n1578 = Insert Into Array(array=w3996, new element=w3995) -> (w3989:i32[])  [unwired: 1 in]
                    n1579 = Insert Into Array(array=w3985, new element=w3986) -> (w3984:i32[])  [unwired: 1 in]
                    n1580 = call "数值二进制转十进制-8.6.vi"("子数组"=w3989) -> ("十进制数值"=w3994:i32)  [unwired: 4 out]
                    n1581 = call "数值二进制转十进制-8.6.vi"("子数组"=w3984) -> ("十进制数值"=w3983:i32)  [unwired: 4 out]
                  }
                  frame Enabled {
                    w4002 = 255 ("高字节1")
                  }
                }
                n1582 = Build Array(w3981, w3979) -> (w3982:i32[])
              }
            }
            n1583 = Insert Into Array(array=w3787, new element=w3788) -> (w3786:dbl[])  [unwired: 1 in]
          }
          n1584 = Build Array(w3783) -> (w3782:dbl[][])
          n1585 = Build Array("一级故障阀值") -> (w3773:string[])
        }
        frame "整组温度不均衡(2)" {
          n1586 = Unbundle By Name(w4008) -> ("一级故障 2"=w4009:refnum<vi>)
          n1587 = property class="Clust (严格)"(reference=w4009) -> ("Value"=w4007:T4)  [unwired: 1 in, 2 out]
          n1588 = for {
            N: 17 -> [_]
            tunnel: w4007 -> [w4019]
            shift-right: [w4016] -> w4013
            shift-left: dbl[] [] -> [w4017]
            i -> [w4020]
            n1589 = case shown="11" w4020 {
              tunnel: w4019 -> [w4021 w4032 w4043 w4053 w4063 w4072 w4084 w4096 w4108 w4120 w4132 w4144 w4158 w4180 w4192 w4201 w4210]
              tunnel: [w4022 w4033 w4044 w4054 w4064 w4074 w4086 w4098 w4110 w4122 w4134 w4145 w4167 w4183 w4191 w4200 w4212] -> w4018
              frame 0, Default {
                # "总电压过高"
                n1590 = disable-structure shown="启用" {
                  disable-tunnel: [w4028 w4031] -> w4024
                  disable-tunnel: [w4027 w4031] -> w4023
                  disable-tunnel: w4021 -> [w4026 _]
                  frame Disabled {
                    n1591 = Unbundle By Name(w4026) -> ("总电压过高"=w4025:dbl)
                    n1592 = call "输入分辨率计算-EV05.vi"("1字节?"=FALSE, "数值"=w4025, "分辨率"=0.1) -> ("低字节"=w4028:dbl, "高字节1"=w4027:dbl)  [unwired: 2 in, 5 out]
                  }
                  frame Enabled {
                    w4031 = 255 ("高字节1")
                  }
                }
                n1593 = Build Array(w4023, w4024) -> (w4022:i32[])
              }
              frame 1 {
                # "总电压过低"
                n1594 = disable-structure shown="启用" {
                  disable-tunnel: [w4039 w4042] -> w4035
                  disable-tunnel: [w4038 w4042] -> w4034
                  disable-tunnel: w4032 -> [w4037 _]
                  frame Disabled {
                    n1595 = Unbundle By Name(w4037) -> ("总电压过低"=w4036:dbl)
                    n1596 = call "输入分辨率计算-EV05.vi"("1字节?"=FALSE, "数值"=w4036, "分辨率"=0.1) -> ("低字节"=w4039:dbl, "高字节1"=w4038:dbl)  [unwired: 2 in, 5 out]
                  }
                  frame Enabled {
                    w4042 = 255 ("高字节1")
                  }
                }
                n1597 = Build Array(w4034, w4035) -> (w4033:i32[])
              }
              frame 2 {
                # "温度过高"
                n1598 = disable-structure shown="启用" {
                  disable-tunnel: [w4049 255 ("高字节1")] -> w4045
                  disable-tunnel: w4043 -> [w4047 _]
                  frame Disabled {
                    n1599 = Unbundle By Name(w4047) -> ("温度过高"=w4046:dbl)
                    n1600 = call "输入分辨率计算-EV05.vi"("1字节?"=TRUE, "数值"=w4046, "偏移量"=-40.0, "分辨率"=1.0) -> ("高字节1"=w4049:dbl)  [unwired: 1 in, 6 out]
                  }
                  frame Enabled {
                  }
                }
                n1601 = Build Array(w4045) -> (w4044:i32[])
              }
              frame 3 {
                # "温度过低"
                n1602 = disable-structure shown="启用" {
                  disable-tunnel: [w4059 255 ("高字节1")] -> w4055
                  disable-tunnel: w4053 -> [w4057 _]
                  frame Disabled {
                    n1603 = Unbundle By Name(w4057) -> ("温度过低"=w4056:dbl)
                    n1604 = call "输入分辨率计算-EV05.vi"("1字节?"=TRUE, "数值"=w4056, "偏移量"=-40.0, "分辨率"=1.0) -> ("高字节1"=w4059:dbl)  [unwired: 1 in, 6 out]
                  }
                  frame Enabled {
                  }
                }
                n1605 = Build Array(w4055) -> (w4054:i32[])
              }
              frame 4 {
                # "整组温度不均衡"
                n1606 = disable-structure shown="启用" {
                  disable-tunnel: [w4068 255 ("高字节1")] -> w4065
                  disable-tunnel: w4063 -> [w4067 _]
                  frame Enabled {
                    n1607 = Unbundle By Name(w4067) -> ("整组温度不均衡"=w4066:dbl)
                    n1608 = call "输入分辨率计算-EV05.vi"("1字节?"=TRUE, "数值"=w4066, "分辨率"=1.0) -> ("高字节1"=w4068:dbl)  [unwired: 2 in, 6 out]
                  }
                  frame Disabled {
                  }
                }
                n1609 = Build Array(w4065) -> (w4064:dbl[])
              }
              frame 5 {
                # "单组电压不均衡"
                n1610 = disable-structure shown="启用" {
                  disable-tunnel: [w4080 w4083] -> w4075
                  disable-tunnel: [w4078 w4083] -> w4073
                  disable-tunnel: w4072 -> [w4077 _]
                  frame Disabled {
                    n1611 = Unbundle By Name(w4077) -> ("单组电压不均衡"=w4076:dbl)
                    n1612 = call "输入分辨率计算-EV05.vi"("1字节?"=FALSE, "数值"=w4076, "偏移量"=0.0, "分辨率"=0.001) -> ("低字节"=w4078:dbl, "高字节1"=w4080:dbl)  [unwired: 1 in, 5 out]
                  }
                  frame Enabled {
                    w4083 = 255 ("高字节1")
                  }
                }
                n1613 = Build Array(w4075, w4073) -> (w4074:i32[])
              }
              frame 6 {
                # "整组电压不均衡"
                n1614 = disable-structure shown="启用" {
                  disable-tunnel: [w4092 w4095] -> w4087
                  disable-tunnel: [w4090 w4095] -> w4085
                  disable-tunnel: w4084 -> [w4089 _]
                  frame Disabled {
                    n1615 = Unbundle By Name(w4089) -> ("整组电压不均衡"=w4088:dbl)
                    n1616 = call "输入分辨率计算-EV05.vi"("1字节?"=FALSE, "数值"=w4088, "偏移量"=0.0, "分辨率"=0.001) -> ("低字节"=w4090:dbl, "高字节1"=w4092:dbl)  [unwired: 1 in, 5 out]
                  }
                  frame Enabled {
                    w4095 = 255 ("高字节1")
                  }
                }
                n1617 = Build Array(w4087, w4085) -> (w4086:i32[])
              }
              frame 7 {
                # "单体电压过高"
                n1618 = disable-structure shown="启用" {
                  disable-tunnel: [w4104 w4107] -> w4099
                  disable-tunnel: [w4102 w4107] -> w4097
                  disable-tunnel: w4096 -> [w4101 _]
                  frame Disabled {
                    n1619 = Unbundle By Name(w4101) -> ("单体电压过高"=w4100:dbl)
                    n1620 = call "输入分辨率计算-EV05.vi"("1字节?"=FALSE, "数值"=w4100, "偏移量"=0.0, "分辨率"=0.001) -> ("低字节"=w4102:dbl, "高字节1"=w4104:dbl)  [unwired: 1 in, 5 out]
                  }
                  frame Enabled {
                    w4107 = 255 ("高字节1")
                  }
                }
                n1621 = Build Array(w4099, w4097) -> (w4098:i32[])
              }
              frame 8 {
                # "单体电压过低"
                n1622 = disable-structure shown="启用" {
                  disable-tunnel: [w4116 w4119] -> w4111
                  disable-tunnel: [w4114 w4119] -> w4109
                  disable-tunnel: w4108 -> [w4113 _]
                  frame Disabled {
                    n1623 = Unbundle By Name(w4113) -> ("单体电压过低"=w4112:dbl)
                    n1624 = call "输入分辨率计算-EV05.vi"("1字节?"=FALSE, "数值"=w4112, "偏移量"=0.0, "分辨率"=0.001) -> ("低字节"=w4114:dbl, "高字节1"=w4116:dbl)  [unwired: 1 in, 5 out]
                  }
                  frame Enabled {
                    w4119 = 255 ("高字节1")
                  }
                }
